vi "Flush LogMeasData Q.vi"(8 "error in (no error)":errorcluster) -> (0 "error out":errorcluster, 1 "Remaining MeasData[] out":T1[](array[typedef]), 3 "orData out":T2)   [LabVIEW 2017]
doc: "Developed by Kevin Thompson\nThompson Engineering, LLC\nkevin@thompsonengineering.net"
uses:
  TD MeasData QRef.ctl
  TD MeasData--cluster.ctl
  GBL DataQ Ref.vi
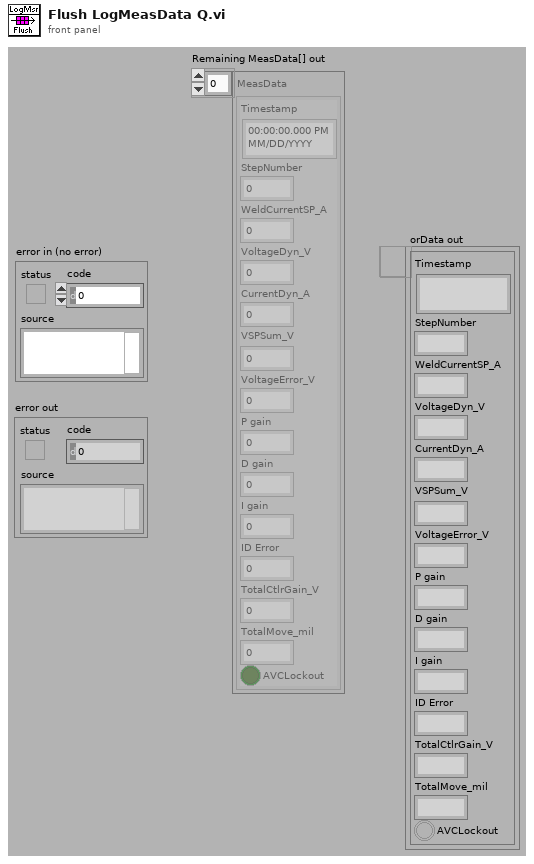
[diagram p1: front panel]
types:
  T1 = typedef "TD MeasData--cluster.ctl" = cluster{"Timestamp":timestamp, "StepNumber":i32, "WeldCurrentSP_A":dbl, "VoltageDyn_V":dbl, "CurrentDyn_A":dbl, "VSPSum_V":dbl, "VoltageError_V":dbl, "P gain":dbl, "D gain":dbl, "I gain":dbl, "ID Error":dbl, "TotalCtlrGain_V":dbl, "TotalMove_mil":dbl, "AVCLockout":bool}
  T2 = typedef "TD MeasData QRef.ctl" = refnum<queue>
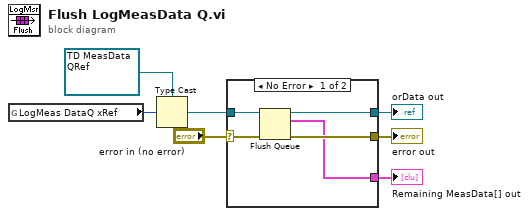
[diagram p0: block diagram]
diagram:
  n1 = global read "GBL DataQ Ref.vi" "LogMeas DataQ xRef"() -> (w1:u32)
  n2 = Type Cast(type=T2 refnum ("MeasDataQRef"), x=w1) -> (*(type *) &x=w4:T2)
  n3 = case shown="No Error" "error in (no error)" {
    selector: "error in (no error)" -> [w9 w13]
    tunnel: w4 -> [w10 w14]
    tunnel: [w12 w13] -> w7
    tunnel: [w11 w14] -> w6
    tunnel: [w8 _] -> w3
    frame No Error {
      n4 = Flush Queue(queue=w10, error in (no error)=w9) -> (queue out=w11:T2, remaining elements=w8:T1[], error out=w12:errorcluster)
    }
    frame Error {
    }
  }
  "orData out" <- w6
  "error out" <- w7
  "Remaining MeasData[] out" <- w3
